vi "Demo2.vi"() -> ()   [LabVIEW 2020, in "VolatusScratch.lvlib"]
uses:
  VolatusScratch.lvlib
  messages/StartLog/Data.ctl
  messages/StartLog/StartLog.lvlib
panel:
  out "Data":T1
  out "Buffer":u8[](array[numeric]) format="%.0x"
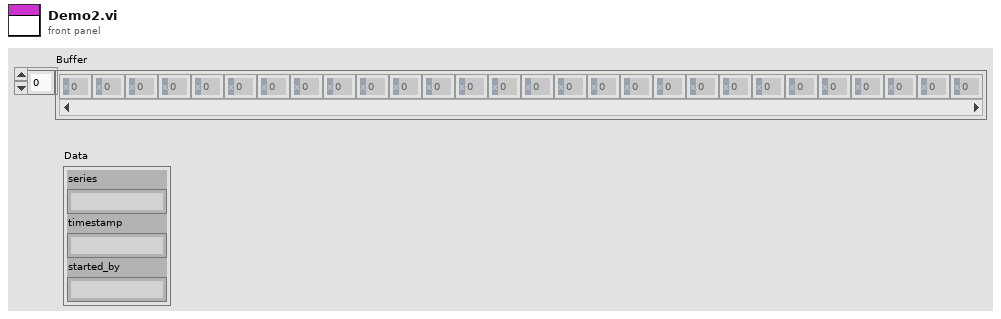
[diagram p1: front panel]
types:
  T1 = typedef "StartLog.lvlib/Data.ctl" = cluster{"series":string, "timestamp":string, "started_by":string}
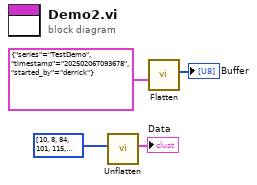
[diagram p0: block diagram]
diagram:
  n1 = call "Unflatten.vi"("Buffer"=u8[] [10, 8, 84, 101, 115, 116, 68, 101, 109, 111, 18, 15, 50, 48, 50, 53, 48, 50, 48, 54, 84, 48, 57, 51, 54, 55, 56]) -> ("Data"=→"Data":T1)  [unwired: 9 in, 1 out]
  n2 = call "Flatten.vi"("Data"=T1 {"series"="TestDemo", "timestamp"="20250206T093678", "started_by"="derrick"} ("StartLog")) -> ("Buffer"=→"Buffer":u8[])  [unwired: 9 in, 1 out]
